vi "NI-DCPower Specific Logic.vi"(7 "connections":T1[](array[typedef]), 8 "error in":errorcluster, 9 "channel list":string, 10 "instrument handle":refnum<k15>, 11 "Measurement Configuration":T4={"pin_names"=[], "voltage_level"=6.0, "voltage_level_range"=6.0, "current_limit"=0.01, "current_limit_range"=0.01, "source_delay"=0.0}) -> (0 "error out":errorcluster, 2 "instrument handle out":refnum<k15>, 3 "Measurement Results":T3)   [LabVIEW 2020, in "NIDCPowerSourceDCVoltage.lvlib"]
uses:
  NIDCPowerSourceDCVoltage.lvlib
  Measurement Configuration.ctl
  Measurement Results.ctl
  <instrlib>/niDCPower/nidcpower.llb/niDCPower Source Mode.ctl
  <instrlib>/niDCPower/nidcpower.llb/niDCPower Output Function.ctl
  <instrlib>/niDCPower/nidcpower.llb/niDCPower Wait For Event - Event.ctl
  <vilib>/MeasurementLink/MeasurementLink Session Management/Session Reservation/Connection.ctl
  <vilib>/MeasurementLink/MeasurementLink Session Management/Session Reservation/Session Reservation.lvclass
  <vilib>/MeasurementLink/MeasurementLink niDCPower/Connection with Session.ctl
  <vilib>/MeasurementLink/MeasurementLink niDCPower/MeasurementLink niDCPower.lvlib
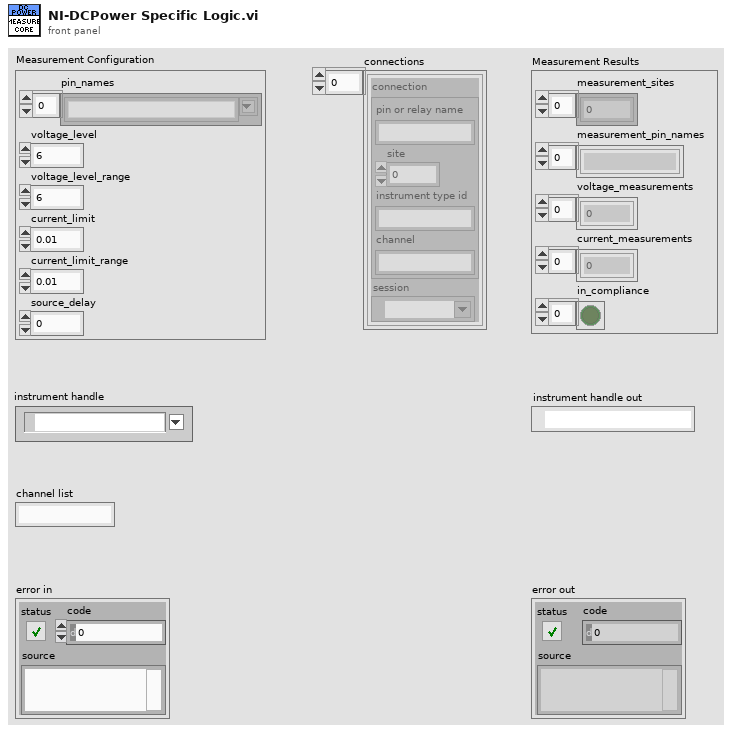
[diagram p1: front panel]
types:
  T1 = typedef "MeasurementLink niDCPower.lvlib/Connection with Session.ctl" = cluster{"connection":T2, "session":refnum<k15>}
  T2 = typedef "MeasurementLink Session Management.lvlib/Session Reservation.lvclass/Connection.ctl" = cluster{"pin or relay name":string, "site":i32, "instrument type id":string, "channel":string}
  T3 = typedef "NIDCPowerSourceDCVoltage.lvlib/Measurement Results.ctl" = cluster{"measurement_sites":i32[], "measurement_pin_names":string[], "voltage_measurements":dbl[], "current_measurements":dbl[], "in_compliance":bool[]}
  T4 = typedef "NIDCPowerSourceDCVoltage.lvlib/Measurement Configuration.ctl" = cluster{"pin_names":string[], "voltage_level":dbl, "voltage_level_range":dbl, "current_limit":dbl, "current_limit_range":dbl, "source_delay":dbl}
  T5 = typedef "niDCPower Wait For Event - Event.ctl" = i32
  T6 = typedef "niDCPower Output Function.ctl" = i32
  T7 = typedef "niDCPower Source Mode.ctl" = i32
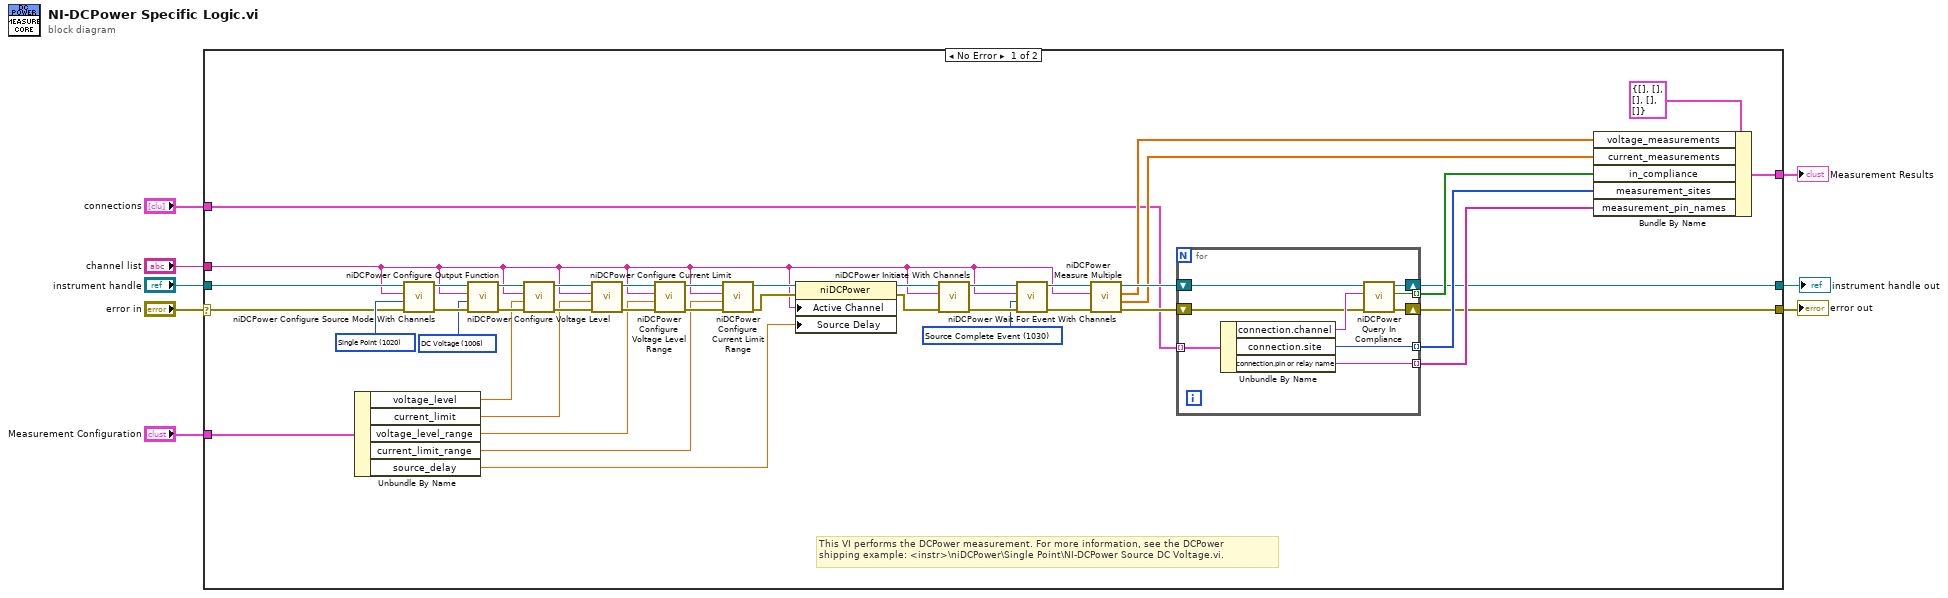
[diagram p0: block diagram]
diagram:
  n1 = case shown="No Error" "error in" {
    selector: "error in" -> [w11 w60]
    tunnel: "Measurement Configuration" -> [w27 _]
    tunnel: [w22 _] -> w7
    tunnel: [w14 w60] -> w6
    tunnel: "instrument handle" -> [w13 w61]
    tunnel: [w12 w61] -> w4
    tunnel: "channel list" -> [w10 _]
    tunnel: "connections" -> [w9 _]
    frame No Error {
      w28 = T5 1030 items=["Source Complete Event"=1030, "Measure Complete Event"=1031, "Sequence Iteration Complete Event"=1032, "Sequence Engine Done Event"=1033, "Pulse Complete Event"=1051, "Ready For Pulse Trigger Event"=1052] ("event")
      w31 = T6 1006 items=["DC Voltage"=1006, "DC Current"=1007, "Pulse Voltage"=1049, "Pulse Current"=1050] ("output function")
      w32 = T7 1020 items=["Single Point"=1020, "Sequence"=1021] ("source mode")
      # "This VI performs the DCPower measurement. For more information, see the DCPower\nshipping example: <instr>\\niDCPower\\Single Point\\NI-DCPower Source DC Voltage.vi."
      n2 = Unbundle By Name(w27) -> ("voltage_level"=w30:dbl, "current_limit"=w29:dbl, "voltage_level_range"=w26:dbl, "current_limit_range"=w25:dbl, "source_delay"=w24:dbl)
      n3 = call <instrlib>:"niDCPower Configure Source Mode With Channels.vi"("error in (no error)"=w11, "source mode"=w32, "channel name"=w10, "instrument handle"=w13) -> ("error out"=w48:errorcluster, "instrument handle out"=w47:refnum<k15>)  [unwired: 6 in]
      n4 = call <instrlib>:"niDCPower Configure Output Function.vi"("error in (no error)"=w48, "output function"=w31, "channel name"=w10, "instrument handle"=w47) -> ("error out"=w33:errorcluster, "instrument handle out"=w34:refnum<k15>)  [unwired: 6 out]
      n5 = call <instrlib>:"niDCPower Configure Voltage Level.vi"("error in (no error)"=w33, "voltage level"=w30, "channel name"=w10, "instrument handle"=w34) -> ("error out"=w49:errorcluster, "instrument handle out"=w50:refnum<k15>)  [unwired: 6 out]
      n6 = call <instrlib>:"niDCPower Configure Current Limit.vi"("error in (no error)"=w49, "current limit"=w29, "channel name"=w10, "instrument handle"=w50) -> ("error out"=w46:errorcluster, "instrument handle out"=w45:refnum<k15>)  [unwired: 1 in, 5 out]
      n7 = call <instrlib>:"niDCPower Configure Voltage Level Range.vi"("error in (no error)"=w46, "voltage level range"=w26, "channel name"=w10, "instrument handle"=w45) -> ("error out"=w44:errorcluster, "instrument handle out"=w43:refnum<k15>)  [unwired: 6 out]
      n8 = call <instrlib>:"niDCPower Configure Current Limit Range.vi"("error in (no error)"=w44, "current limit range"=w25, "channel name"=w10, "instrument handle"=w43) -> ("error out"=w39:errorcluster, "instrument handle out"=w42:refnum<k15>)  [unwired: 6 out]
      n9 = property class="niDCPower"(reference=w42, error in=w39, "Active Channel"=w10, "Source Delay"=w24) -> (reference out=w41:refnum<k15>, error out=w40:errorcluster)
      n10 = call <instrlib>:"niDCPower Initiate With Channels.vi"("error in (no error)"=w40, "channel name"=w10, "instrument handle"=w41) -> ("error out"=w36:errorcluster, "instrument handle out"=w38:refnum<k15>)  [unwired: 7 in]
      n11 = call <instrlib>:"niDCPower Wait For Event With Channels.vi"("error in (no error)"=w36, "event"=w28, "channel name"=w10, "instrument handle"=w38) -> ("error out"=w35:errorcluster, "instrument handle out"=w37:refnum<k15>)  [unwired: 6 in]
      n12 = call <instrlib>:"niDCPower Measure Multiple.vi"("error in (no error)"=w35, "channel name"=w10, "instrument handle"=w37) -> ("error out"=w20:errorcluster, "current measurements"=w18:dbl[], "voltage measurements"=w19:dbl[], "instrument handle out"=w21:refnum<k15>)  [unwired: 5 out]
      n13 = for {
        tunnel: w9 -> [w59] mode=indexing
        tunnel: [w58] -> w16 mode=indexing
        tunnel: [w57] -> w15 mode=indexing
        shift-right: [w54] -> w12
        shift-left: w21 -> [w55]
        shift-right: [w52] -> w14
        shift-left: w20 -> [w53]
        tunnel: [w51] -> w17 mode=indexing
        n14 = Unbundle By Name(w59) -> ("connection.channel"=w56:string, "connection.site"=w58:i32, "connection.pin or relay name"=w57:string)
        n15 = call <instrlib>:"niDCPower Query In Compliance.vi"("error in (no error)"=w53, "channel name"=w56, "instrument handle"=w55) -> ("error out"=w52:errorcluster, "in compliance?"=w51:bool, "instrument handle out"=w54:refnum<k15>)  [unwired: 6 out]
      }
      n16 = Bundle By Name(cluster=T3 {"measurement_sites"=[], "measurement_pin_names"=[], "voltage_measurements"=[], "current_measurements"=[], "in_compliance"=[]} ("Measurement Results"), "voltage_measurements"=w19, "current_measurements"=w18, "in_compliance"=w17, "measurement_sites"=w16, "measurement_pin_names"=w15) -> (w22:T3)
    }
    frame Error {
    }
  }
  "Measurement Results" <- w7
  "error out" <- w6
  "instrument handle out" <- w4
